vi "test_fmcw.vi"() -> ()   [LabVIEW 2020]
uses:
  <vilib>/Platform/storage/Storage.llb/usiSequenceRepresentation.ctl
  <extravilib>/ChannelInstances/Stream-bool/Read With Abort.vi
  <extravilib>/ChannelInstances/Stream-a[.](sgl)/Read With Abort.vi
  <extravilib>/ChannelInstances/Stream-a[.](sgl)/Write With Abort.vi
  <extravilib>/ChannelInstances/Stream-bool/Write With Abort.vi
  <extravilib>/ChannelInstances/Stream-bool/EndpointRead.vi
  <extravilib>/ChannelInstances/Stream-a[.](sgl)/EndpointRead.vi
  <extravilib>/ChannelInstances/Stream-a[.](sgl)/Endpoint.vi
  <extravilib>/ChannelInstances/Stream-bool/Endpoint.vi
  <vilib>/Platform/storage/lvStorage.llb/_openStorageWithRootAutoDetect.vi
  <vilib>/Platform/storage/lvStorage.llb/xStorage/xStorageSupp/ErrorOut.vi
  <extravilib>/ChannelInstances/Stream-bool/Instantiate.vi
  <extravilib>/ChannelInstances/Stream-a[.](sgl)/Instantiate.vi
  <extravilib>/ChannelInstances/Stream-bool/)Channel.vi
  <resource>/ChannelSupport/_ChannelSupport/WaitIfNeeded.vi
  <extravilib>/ChannelInstances/Stream-a[.](sgl)/)Channel.vi
  <vilib>/Platform/storage/lvStorage.llb/_createOrGetExplicitChildObject.vi
  <vilib>/Platform/storage/lvStorage.llb/_createOrGetByNameExplicitChildObject.vi
  <vilib>/Platform/storage/lvStorage.llb/_saveFloat32Channel.vi
  <vilib>/Platform/storage/Storage.llb/Get Object Info.vi
  <vilib>/Platform/storage/Storage.llb/__closeStorageFromObject.vi
  <vilib>/Platform/storage/lvStorage.llb/xStorage/Open Data Storage/Open Data Storage.xnode
  <vilib>/Platform/storage/lvStorage.llb/xStorage/Write Data/Write Data.xnode
  <vilib>/Platform/storage/lvStorage.llb/xStorage/Close Data Storage/Close Data Storage.xnode
  <extravilib>/ChannelInstances/Stream-a[.](sgl).lvlib
  <extravilib>/ChannelInstances/Stream-bool.lvlib
panel:
  out "AiFifoUsed":i32
  in  "set_time(s)":u64=10 min=10 max=120
  in  "AiSampleRate":u32(ring)=2000 items=["100K"=10000, "250K"=4000, "500K"=2000]
  out "time":dbl
  in  "stop":bool
  out "error out":errorcluster caption="错误输出"
  out "波形图":sgl[][](graph)
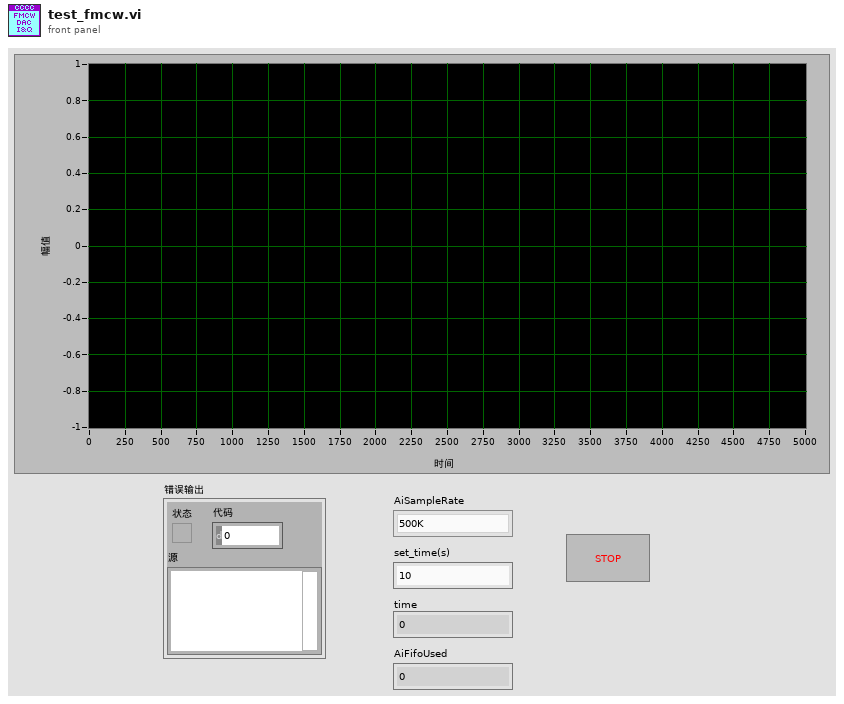
[diagram p1: front panel]
types:
  T1 = enum16{"open", "open or create", "create or replace", "create", "open (read only)"}
  T2 = enum8{"Enabled", "Disabled", "Disabled and Grayed Out"}
  T3 = typedef "Stream-a[.](sgl).lvlib/)Channel.ctl" = refnum<queue>
  T4 = typedef "Stream-bool.lvlib/)Channel.ctl" = refnum<queue>
  T5 = enum16{"Append values", "Replace values at index", "Replace all values"}
  T6 = enum16{"UPDATE", "READ", "QUERY", "CREATE CHILD", "CREATE", "CONNECT", "DISCONNECT"}
  T7 = typedef "usiSequenceRepresentation.ctl" = enum16{"explicit", "implicit"}
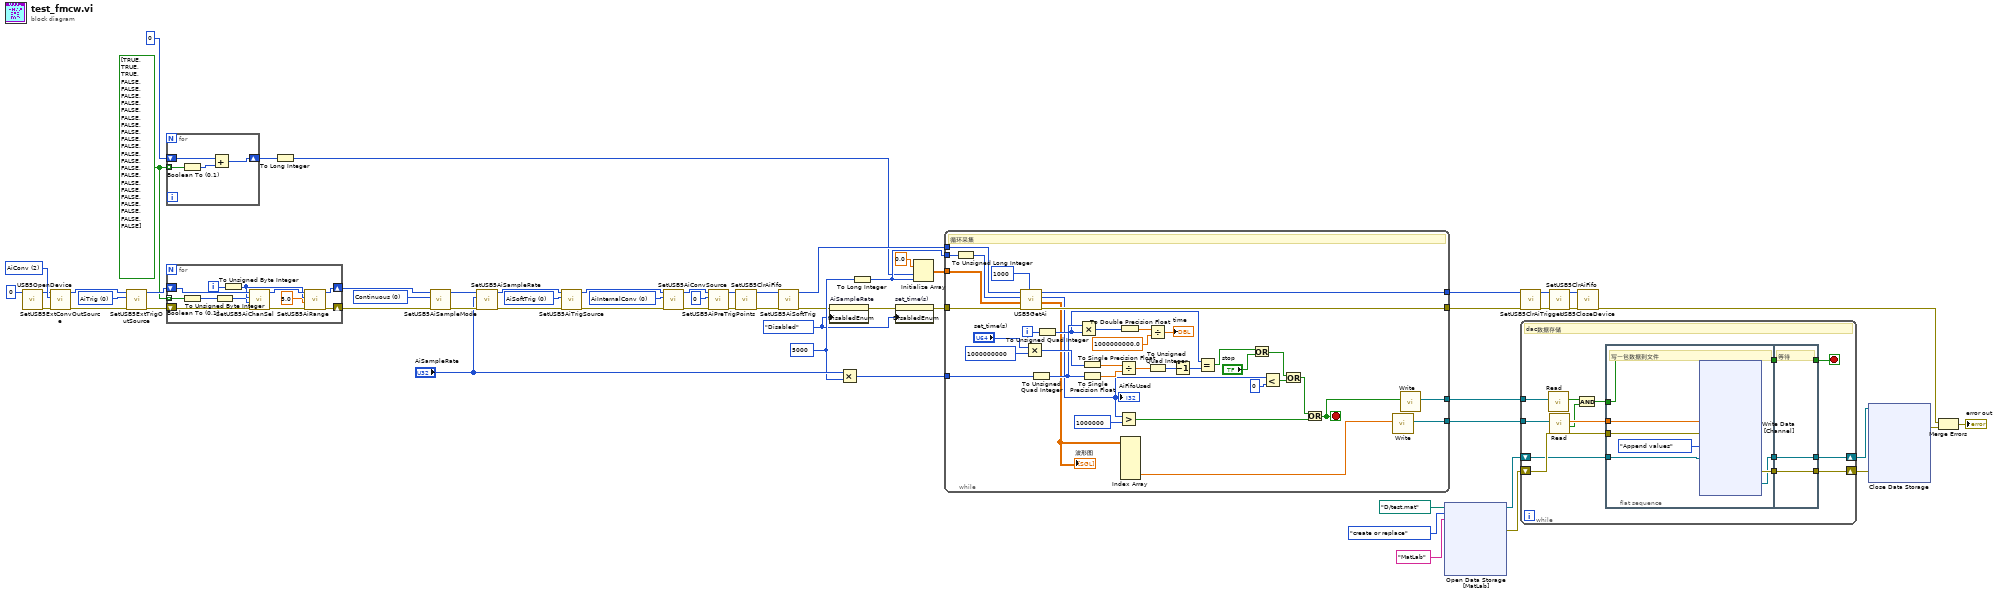
[diagram p0: block diagram]
diagram:
  w16 = T2."Disabled" ("Disabled")
  w25 = bool[] [TRUE, TRUE, TRUE, FALSE, FALSE, FALSE, FALSE, FALSE, FALSE, FALSE, FALSE, FALSE, FALSE, FALSE, FALSE, FALSE, FALSE, FALSE, FALSE, FALSE, FALSE, FALSE, FALSE, FALSE] ("ChanSel")
  w20 = u32 5000 ("number")
  w41 = u8 0 items=["AiInternalConv"=0, "ConvIn"=1, "DiConv"=3, "DoConv"=4, "Ao0Conv"=5, "Ao1Conv"=6, "Ao2Conv"=7, "Ao3Conv"=8] ("AiConvSource")
  w44 = u8 0 items=["AiSoftTrig"=0, "ExtTrigIn"=1, "Din0RisingEdge"=2, "Din1RisingEdge"=3, "Din2RisingEdge"=4, "Din3RisingEdge"=5, "WithDiTrig"=7, "WithDoTrig"=8, "WithAo0Trig"=9, "WithAo1Trig"=10, "WithAo2Trig"=11, "WithAo3Trig"=12, "GlobalSoftTrig"=255] ("AiTrigSource")
  w49 = u8 0 items=["Continuous", "OneShot"] ("AiSampleMode")
  w54 = u8 0 items=["AiTrig", "DiTrig", "DoTrig", "Ao0Trig", "Ao1Trig", "Ao2Trig", "Ao3Trig"] ("Source")
  w59 = u8 2 items=["AiConv"=2, "DiConv"=3, "DoConv"=4, "Ao0Conv"=5, "Ao1Conv"=6, "Ao2Conv"=7, "Ao3Conv"=8] ("Source")
  n1 = call "USB5OpenDevice.vi"("DevIndex"=0) -> ("error out"=w57:errorcluster, "DevIndex Out"=w58:i32)  [unwired: 9 in]
  n2 = call "SetUSB5ExtConvOutSource.vi"("错误输入（无错误）"=w57, "Source"=w59, "DevIndex"=w58) -> ("错误输出"=w56:errorcluster, "DevIndex Out"=w55:i32)  [unwired: 7 in]
  n3 = call "SetUSB5ExtTrigOutSource.vi"("错误输入（无错误）"=w56, "Source"=w54, "DevIndex"=w55) -> ("错误输出"=w52:errorcluster, "DevIndex Out"=w53:i32)  [unwired: 7 in]
  n4 = for {
    tunnel: w25 -> [w64] mode=indexing
    shift-right: [w61] -> w23
    shift-left: i16 0 -> [w62]
    n5 = Boolean To (0,1)(Boolean=w64) -> (0, 1=w63:i16)
    n6 = Add(x=w62, y=w63) -> (x+y=w61:i16)
  }
  n7 = for {
    shift-right: [w71] -> w50
    shift-left: w53 -> [w75]
    shift-right: [w70] -> w51
    shift-left: w52 -> [w74]
    tunnel: w25 -> [w67] mode=indexing
    i -> [w76]
    n8 = Boolean To (0,1)(Boolean=w67) -> (0, 1=w66:i16)
    n9 = To Unsigned Byte Integer(number=w66) -> (unsigned 8bit integer=w65:u8)
    n10 = To Unsigned Byte Integer(number=w76) -> (unsigned 8bit integer=w69:u8)
    n11 = call "SetUSB5AiChanSel.vi"("错误输入（无错误）"=w74, "Sel"=w65, "Chan"=w69, "DevIndex"=w75) -> ("错误输出"=w73:errorcluster, "DevIndex Out"=w72:i32)  [unwired: 6 in]
    n12 = call "SetUSB5AiRange.vi"("错误输入（无错误）"=w73, "AiRange"=sgl 5.0, "Chan"=w69, "DevIndex"=w72) -> ("错误输出"=w70:errorcluster, "DevIndex Out"=w71:i32)  [unwired: 6 in]
  }
  n13 = To Long Integer(number=w23) -> (32bit integer=w22:i32)
  n14 = call "SetUSB5AiSampleMode.vi"("错误输入（无错误）"=w51, "AiSampleMode"=w49, "DevIndex"=w50) -> ("错误输出"=w47:errorcluster, "DevIndex Out"=w48:i32)  [unwired: 7 in]
  n15 = call "SetUSB5AiSampleRate.vi"("错误输入（无错误）"=w47, "SamplePeriod(ns)"="AiSampleRate", "DevIndex"=w48) -> ("错误输出"=w46:errorcluster, "DevIndex Out"=w45:i32)  [unwired: 7 in]
  n16 = call "SetUSB5AiTrigSource.vi"("错误输入（无错误）"=w46, "AiTrigSource"=w44, "DevIndex"=w45) -> ("错误输出"=w43:errorcluster, "DevIndex Out"=w42:i32)  [unwired: 7 in]
  n17 = call "SetUSB5AiConvSource.vi"("错误输入（无错误）"=w43, "AiConvSource"=w41, "DevIndex"=w42) -> ("错误输出"=w40:errorcluster, "DevIndex Out"=w38:i32)  [unwired: 7 in]
  n18 = call "SetUSB5AiPreTrigPoints.vi"("错误输入（无错误）"=w40, "AiPreTrigPoints"=u32 0, "DevIndex"=w38) -> ("错误输出"=w36:errorcluster, "DevIndex Out"=w37:i32)  [unwired: 7 in]
  n19 = call "SetUSB5ClrAiFifo.vi"("错误输入（无错误）"=w36, "DevIndex"=w37) -> ("错误输出"=w34:errorcluster, "DevIndex Out"=w35:i32)  [unwired: 8 in]
  n20 = call "SetUSB5AiSoftTrig.vi"("错误输入（无错误）"=w34, "DevIndex"=w35) -> ("错误输出"=w18:errorcluster, "DevIndex Out"=w32:i32)  [unwired: 8 in]
  n21 = property on="AiSampleRate" class="Ring (strict)"(error in=w18, "DisabledEnum"=w16) -> (error out=w17:errorcluster)  [unwired: 1 in, 1 out]
  n22 = Multiply(x="AiSampleRate", y=w20) -> (x*y=w19:u32)
  n23 = To Long Integer(number=w20) -> (32bit integer=w26:i32)
  n24 = property on="set_time(s)" class="DigNum (strict)"(error in=w17, "DisabledEnum"=w16) -> (error out=w11:errorcluster)  [unwired: 1 in, 1 out]
  n25 = Initialize Array(sgl 0.0 ("element"), w22, w26) -> (w31:sgl[][])
  n26 = while {
    tunnel: w26 -> [w109]
    tunnel: w31 -> [w110]
    tunnel: w11 -> [w113]
    tunnel: w32 -> [w114]
    tunnel: [w112] -> w13
    tunnel: w19 -> [w101]
    tunnel: [w87] -> w12
    tunnel: [w78] -> w10
    tunnel: [w77] -> w8
    i -> [w107]
    stop <- w81 stop-if-true
    # "循环采集"
    n27 = To Unsigned Long Integer(number=w109) -> (unsigned 32bit integer=w108:u32)
    n28 = call "USB5GetAi.vi"("TimeOut"=1000, "错误输入（无错误）"=w113, "Ai"=w110, "Points"=w108, "DevIndex"=w114) -> ("错误输出"=w87:errorcluster, "Ai Out"=w86:sgl[][], "AiFifoUsed"=w85:i32, "DevIndex Out"=w112:i32)  [unwired: 3 in]
    "波形图" <- w86
    "AiFifoUsed" <- w85
    n29 = Multiply(x="set_time(s)", y=u64 1000000000) -> (x*y=w97:u64)
    n30 = To Unsigned Quad Integer(1:w101) -> (0:w95:u64)
    n31 = To Unsigned Quad Integer(1:w107) -> (0:w91:u64)
    n32 = Multiply(x=w95, y=w91) -> (x*y=w100:u64)
    n33 = To Single Precision Float(number=w97) -> (single precision float=w96:sgl)
    n34 = To Single Precision Float(number=w95) -> (single precision float=w94:sgl)
    n35 = Divide(x=w96, y=w94) -> (x/y=w93:sgl)
    n36 = Greater?(x=w85, y=1000000) -> (0:w82:bool)
    n37 = To Double Precision Float(number=w100) -> (double precision float=w88:dbl)
    n38 = Index Array(array=w86) -> (element #3=w79:sgl[])  [unwired: 6 in, 2 out]
    n39 = Divide(x=w88, y=1000000000.0) -> (x/y=→"time":dbl)
    n40 = To Unsigned Quad Integer(1:w93) -> (0:w92:u64)
    n41 = Decrement(x=w92) -> (x-1=w80:u64)
    n42 = Equal?(x=w91, y=w80) -> (x = y?=w106:bool)
    n43 = Or(x=w106, y="stop") -> (x .or. y?=w102:bool)
    n44 = Less?(x=w85, y=0) -> (x < y?=w103:bool)
    n45 = Or(x=w102, y=w103) -> (x .or. y?=w83:bool)
    n46 = Or(x=w83, y=w82) -> (x .or. y?=w81:bool)
    n47 = call <extravilib>:"Write.vi"("element"=w79) -> ("channel"=w78:T3)  [unwired: 8 in, 2 out]
    n48 = call <extravilib>:"Write.vi"("element"=w81) -> ("channel"=w77:T4)  [unwired: 8 in, 2 out]
  }
  n49 = xnode "Open Data Storage\n[MatLab]"("file path"=path "D:/test.mat", "function (open:0)"=T1."create or replace", "DataPlugin name"="MatLab") -> ("storage refnum (file)"=w5:refnum<k20>, "error out"=w9:errorcluster)  [unwired: 2 in, 1 out]
  n50 = call "SetUSB5ClrAiTrigger.vi"("错误输入（无错误）"=w12, "DevIndex"=w13) -> ("错误输出"=w27:errorcluster, "DevIndex Out"=w30:i32)  [unwired: 8 in]
  n51 = while {
    tunnel: w10 -> [w128]
    tunnel: w8 -> [w125]
    shift-right: [w123] -> w6
    shift-left: w5 -> [w122]
    shift-right: [w124] -> w7
    shift-left: w9 -> [w126]
    stop <- w115 stop-if-true
    # "dac数据存储"
    n52 = call <extravilib>:"Read.vi"("channel"=w125) -> ("element"=w121:bool)  [unwired: 6 in, 4 out]
    n53 = call <extravilib>:"Read.vi"("channel"=w128) -> ("last element?"=w120:bool, "element"=w127:sgl[])  [unwired: 6 in, 3 out]
    n54 = And(x=w121, y=w120) -> (x .and. y?=w117:bool)
    n55 = flat-sequence {
      tunnel: w127 -> [w134]
      tunnel: w126 -> [w133]
      tunnel: w122 -> [w130]
      tunnel: [w132] -> w119
      tunnel: [w131] -> w118
      tunnel: w117 -> [w129]
      tunnel: [w129] -> w116
      tunnel: [w158] -> w123
      tunnel: [w159] -> w124
      tunnel: w119 -> [w159]
      tunnel: w118 -> [w158]
      tunnel: w116 -> [w157]
      tunnel: [w157] -> w115
      frame #0 {
        # "写一包数据到文件"
        n56 = xnode "Write Data\n[Channel]"("Signal"=w134, "error in"=w133, "append / replace (append data values)"=T5."Append values", "storage refnum (file)"=w130) -> ("error out"=w132:errorcluster, "storage refnum (file) out"=w131:refnum<k20>)  [unwired: 1 in, 1 out]
      }
      frame #1 {
        # "等待"
      }
    }
  }
  n57 = call "SetUSB5ClrAiFifo.vi"("错误输入（无错误）"=w27, "DevIndex"=w30) -> ("错误输出"=w28:errorcluster, "DevIndex Out"=w29:i32)  [unwired: 8 in]
  n58 = call "USB5CloseDevice.vi"("错误输入（无错误）"=w28, "DevIndex"=w29) -> ("error out"=w4:errorcluster)  [unwired: 8 in, 1 out]
  n59 = xnode "Close Data Storage\n"("error in (no error)"=w7, "storage refnum (file)"=w6) -> ("error out"=w2:errorcluster)  [unwired: 1 out]
  n60 = Merge Errors(w4, w2) -> (→"error out":errorcluster)
